vi "SendAllData.vi"(9 "ListOfSlotsAndOutputs":u8[](array[numeric]), 10 "NewDigitalOutput":u8[](array[numeric]), 11 "MockDigitalOutput":cluster{"BufferUpdateFIFO":refnum<k21>}={"BufferUpdateFIFO"="MockDigitalOutputCommand"}) -> ()   [LabVIEW 2016, in "FPGAMockDigitalOutput.lvlib"]
uses:
  FPGAMockDigitalOutput.lvlib
  <vilib>/rvi/DataTransferAndStorage/Container/Common/niFpgaContainerExecOnDevCompGetState.vi
  <vilib>/rvi/Emulation/niFpgaEmulationIsFPGAContextNoSignature.vi
  <vilib>/rvi/Emulation/niFpgaSctlEmulationGetInTimedLoop.vi
  <vilib>/rvi/errors/niFpgaSetErrorForExecOnDevCompSimple.vi
  <vilib>/rvi/eio/common/nirviEmuReportErrorAndStop.vi
  <vilib>/rvi/DataTransferAndStorage/Container/Common/niFpgaContainerGetUniqueNameForEmu.vi
  <vilib>/rvi/FIFO/Fifo_Resource/nirvififoEmulationSetSize.vi
  <vilib>/rvi/FIFO/Fifo_Resource/nirviFifoEmulationQueueMgr.vi
  <instcachedir>/0/nirviFifoEmulationQueueMgr_E5CAEC123FF24DC58D834DCA3CDAA9B5.lvgen/nirviFifoEmulationQueueMgr_E5CAEC123FF24DC58D834DCA3CDAA9B5_000.vi
  <vilib>/rvi/FIFO/Fifo_Resource/nirvififoEmulationDetermineInputValidOut.vi
  <vilib>/rvi/FIFO/Fifo_Resource/nirvififoEmulationCreateLock.vi
  <vilib>/rvi/Emulation/niFpgaProcessEmulError.vi
  <vilib>/rvi/FIFO/Fifo_Resource/nirvififoEmulationObtainLock.vi
  <vilib>/rvi/FIFO/Fifo_Resource/nirvififoEmulationReleaseLock.vi
  <vilib>/rvi/occurrence/nirviWaitOnOccurrenceBase.vi
  <vilib>/rvi/errors/nirviReportUnexpectedCaseInternalError.vi
  <vilib>/rvi/errors/nirviReportUnexpectedCaseInternalError (U32).vi
  <vilib>/Utility/error.llb/Clear Errors.vi
  <vilib>/rvi/interface/RandomDataEmulation/niFpgaRandomDataHandleErrors.vi
  <vilib>/rvi/DataTransferAndStorage/Container/XNode/niFpgaContainer.xnode
  <vilib>/rvi/FIFO/Fifo_Resource/niFpgaFifoEmulationRefIn.vi
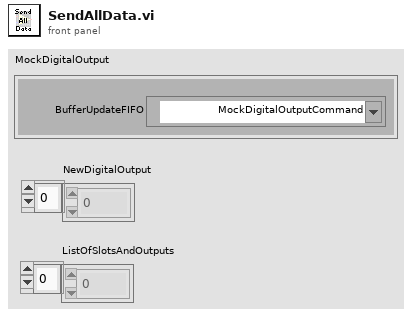
[diagram p1: front panel]
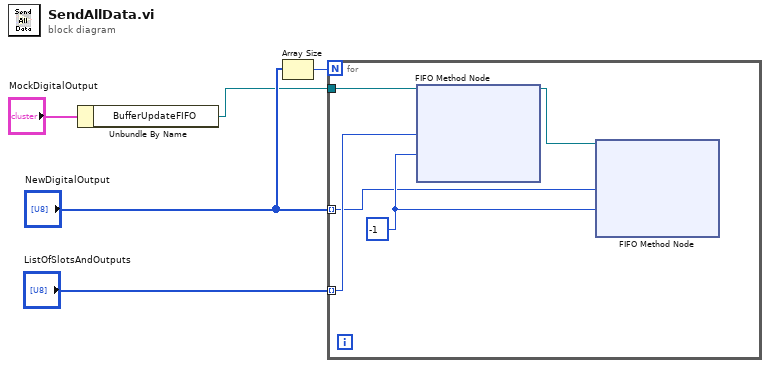
[diagram p0: block diagram]
diagram:
  n1 = Unbundle By Name("MockDigitalOutput") -> ("BufferUpdateFIFO"=w1:refnum<k21>)
  n2 = Array Size(array="NewDigitalOutput") -> (size(s)=w4:i32)
  n3 = for {
    N: w4 -> [_]
    tunnel: "NewDigitalOutput" -> [w6] mode=indexing
    tunnel: "ListOfSlotsAndOutputs" -> [w7] mode=indexing
    tunnel: w1 -> [w8]
    w10 = -1 ("Timeout")
    n4 = xnode ("FIFO Method Node")("Element"=w7, "Timeout"=w10, "FIFO In"=w8) -> ("FIFO Out"=w9:refnum<k21>)  [unwired: 1 out]
    n5 = xnode ("FIFO Method Node")("Element"=w6, "Timeout"=w10, "FIFO In"=w9) -> ()  [unwired: 2 out]
  }
